vi "test JSONPath to EXCEL.vi"(11 "Test Case In":refnum<class "Test Config From EXCEL.lvclass">) -> (0 "error out":errorcluster, 3 "Test Case Out":refnum<class "Test Config From EXCEL.lvclass">)   [LabVIEW 2020, in "Test Config From EXCEL.lvclass"]
uses:
  Test Config From EXCEL.lvclass
  Test Config From EXCEL.lvclass/Test Config From EXCEL.ctl
  <vilib>/Astemes/LUnit/Test Case.lvclass
  Source/Config from EXCEL/Config from EXCEL.lvclass
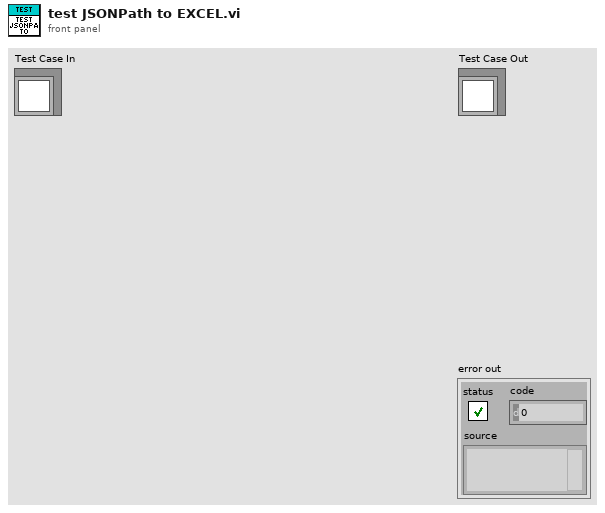
[diagram p1: front panel]
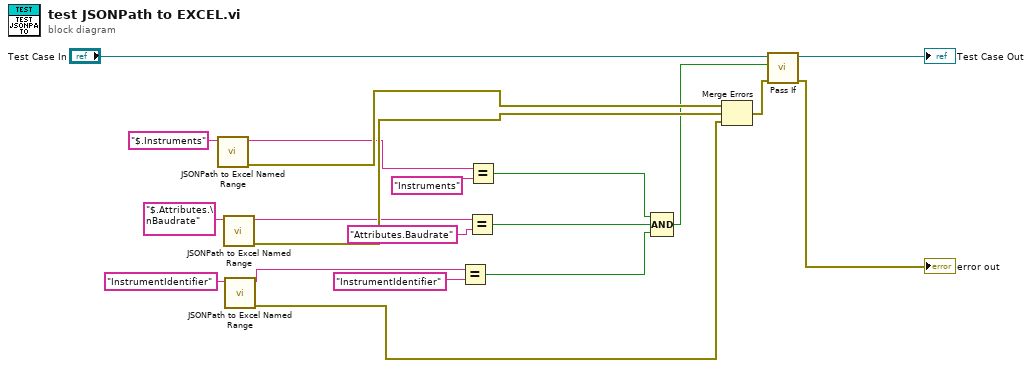
[diagram p0: block diagram]
diagram:
  n1 = call "JSONPath to Excel Named Range.vi"("JSONPath"="$.Instruments") -> ("error out"=w14:errorcluster, "Named Range"=w9:string)  [unwired: 9 in]
  n2 = call "JSONPath to Excel Named Range.vi"("JSONPath"="$.Attributes.\nBaudrate") -> ("error out"=w13:errorcluster, "Named Range"=w7:string)  [unwired: 9 in]
  n3 = call "JSONPath to Excel Named Range.vi"("JSONPath"="InstrumentIdentifier") -> ("error out"=w12:errorcluster, "Named Range"=w5:string)  [unwired: 9 in]
  n4 = Equal?(x=w5, y="InstrumentIdentifier") -> (x = y?=w1:bool)
  n5 = Equal?(x=w7, y="Attributes.Baudrate") -> (x = y?=w2:bool)
  n6 = Equal?(x=w9, y="Instruments") -> (x = y?=w3:bool)
  n7 = Compound Arithmetic op=AND(w3, w2, w1) -> (w10:bool)
  n8 = Merge Errors(w14, w13, w12) -> (w11:errorcluster)
  n9 = call <vilib>:"Pass If.vi"("error in (no error)"=w11, "Pass?"=w10, "LUnit Test Case In"="Test Case In") -> ("error out"=→"error out":errorcluster, "LUnit Test Case Out"=→"Test Case Out":refnum<class "Test Config From EXCEL.lvclass">)  [unwired: 7 in]
